vi "Section Page.vi"(8 "error in (no error)":errorcluster, 11 "Node Ptr":T1 format="%.0x") -> (0 "error out":errorcluster)   [LabVIEW 2019, in "Ghost Bus Addon System Explorer.lvlib"]
uses:
  Ghost Bus Addon System Explorer.lvlib
  <vilib>/NI VeriStand/Custom Device API/Custom Device API.lvlib
  Addon Shared/SubVIs/GUID Lookup.vi
  Addon Shared/Ghost Bus Addon Shared.lvlib
  <vilib>/NI VeriStand/Custom Device API/Custom Device Item Ref.ctl
panel:
  in  "SHDocVw.IWebBrowser2":refnum<k7>(container)
types:
  T1 = typedef "Custom Device API.lvlib/Custom Device Item Ref.ctl" = u64
  T2 = typedef "Custom Device API.lvlib/Custom Device Item Info.ctl" = cluster{"Name":string, "Is Channel":bool, "GUID":string, "Is Waveform":bool}
  T3 = typedef "Custom Device API.lvlib/Custom Device Commands.ctl" = enum16{"Default", "Item renamed", "Shutdown", "Dynamic button pressed"}
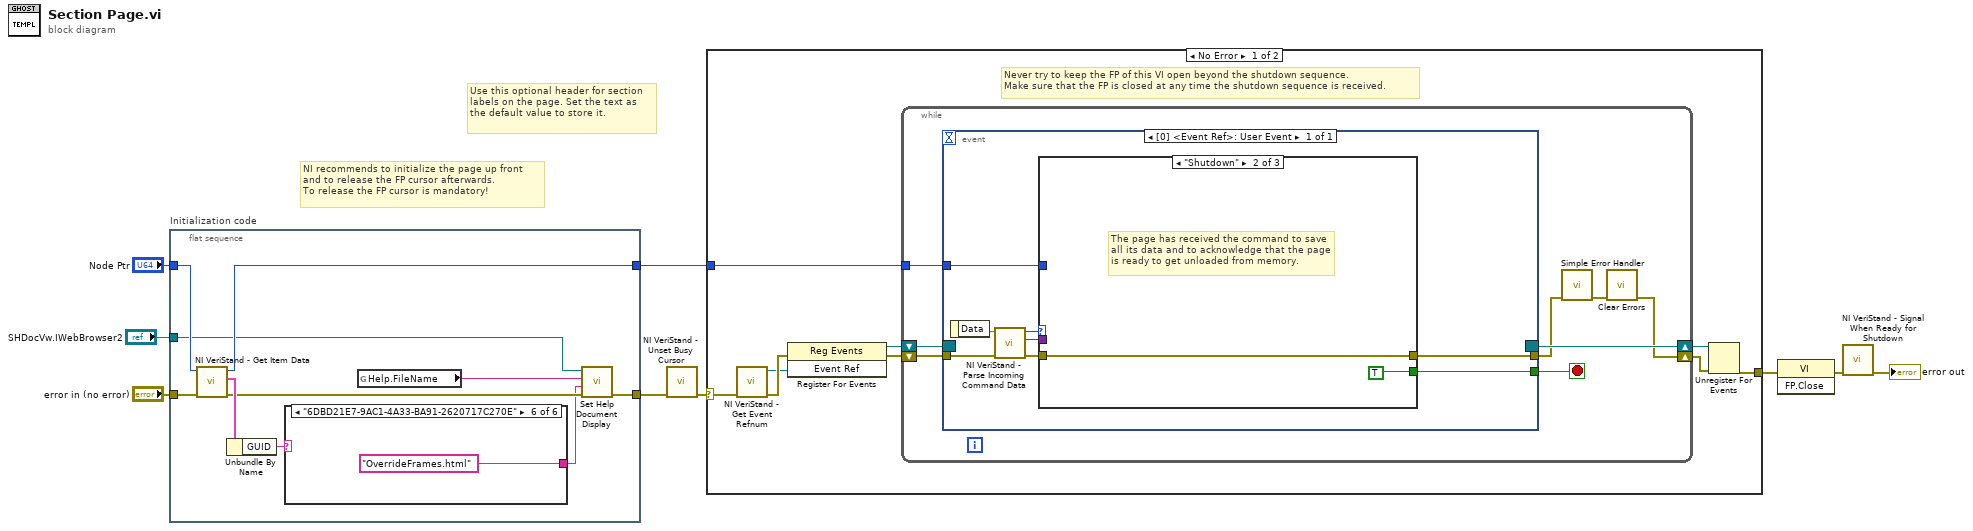
[diagram p0: block diagram]
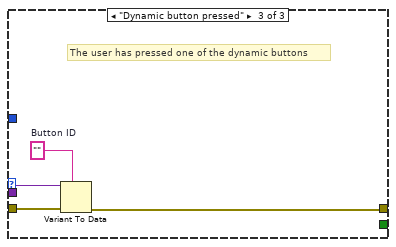
[diagram p3: hidden frame]
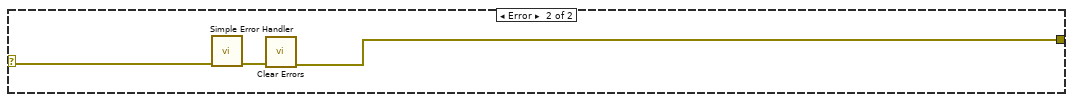
[diagram p4: hidden frame]
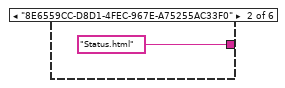
[diagram p6: hidden frame]
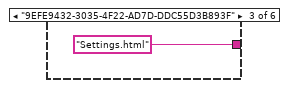
[diagram p7: hidden frame]
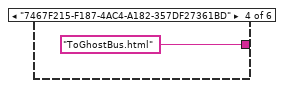
[diagram p8: hidden frame]
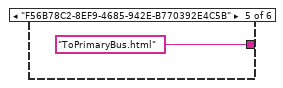
[diagram p9: hidden frame]
diagram:
  # "Use this optional header for section labels on the page. Set the text as the default value to store it."
  # "NI recommends to initialize the page up front\nand to release the FP cursor afterwards.\nTo release the FP cursor is mandatory!"
  n1 = flat-sequence "Initialization code" {
    tunnel: "error in (no error)" -> [w17]
    tunnel: "Node Ptr" -> [w19]
    tunnel: [w13] -> w5
    tunnel: [w18] -> w2
    tunnel: "SHDocVw.IWebBrowser2" -> [w11]
    frame #0 {
      n2 = call <vilib>:"NI VeriStand - Get Item Data.vi"("error in (no error)"=w17, "Item Ref in"=w19) -> ("error out"=w14:errorcluster, "Item Info"=w16:T2, "Item Ref out"=w18:T1)  [unwired: 6 in, 1 out]
      n3 = Unbundle By Name(w16) -> ("GUID"=w15:string)
      n4 = case shown="\"6DBD21E7-9AC1-4A33-BA91-2620717C270E\"" w15 {
        tunnel: [_ "Status.html" ("HTML File") "Settings.html" ("HTML File") "ToGhostBus.html" ("HTML File") "ToPrimaryBus.html" ("HTML File") "OverrideFrames.html" ("HTML File")] -> w12
        frame Default {
        }
        frame "8E6559CC-D8D1-4FEC-967E-A75255AC33F0" {
        }
        frame "9EFE9432-3035-4F22-AD7D-DDC55D3B893F" {
        }
        frame "7467F215-F187-4AC4-A182-357DF27361BD" {
        }
        frame "F56B78C2-8EF9-4685-942E-B770392E4C5B" {
        }
        frame "6DBD21E7-9AC1-4A33-BA91-2620717C270E" {
        }
      }
      n5 = global read "GUID Lookup.vi" "Help.FileName"() -> (w10:string)
      n6 = call "Set Help Document Display.vi"("error in (no error)"=w14, "HTML File"=w12, "Main CHM File"=w10, "SHDocVw.IWebBrowser2"=w11) -> ("error out"=w13:errorcluster)  [unwired: 7 in]
    }
  }
  n7 = call <vilib>:"NI VeriStand - Unset Busy Cursor.vi"("error in (no error)"=w5) -> ("error out"=w4:errorcluster)  [unwired: 10 out]
  n8 = case shown="No Error" w4 {
    selector: w4 -> [w25 w59]
    tunnel: [w30 w57] -> w9
    tunnel: w2 -> [w26 _]
    frame No Error {
      # "Never try to keep the FP of this VI open beyond the shutdown sequence.\nMake sure that the FP is closed at any time the shutdown sequence is received."
      n9 = call <vilib>:"NI VeriStand - Get Event Refnum.vi"("error in (no error)"=w25) -> ("error out"=w33:errorcluster, "Event Ref"=w29:refnum<user-event>)  [unwired: 9 out]
      n10 = register-events(error in=w33, w29) -> (reference out=w27:refnum<event-registration>, error out=w28:errorcluster)  [unwired: 1 in]
      n11 = while {
        tunnel: w26 -> [w37]
        shift-right: [w34] -> w31
        shift-left: w28 -> [w40]
        shift-right: [w41] -> w32
        shift-left: w27 -> [w39]
        stop <- w38 stop-if-true
        n12 = event shown="[0] <Event Ref>: User Event" {
          selector: w39 -> [_]
          dyn-events: [_] -> w41
          timeout: _ -> [_]
          tunnel: w40 -> [w49]
          tunnel: [w45] -> w38
          tunnel: [w44] -> w36
          tunnel: w37 -> [w43]
          event User Event {
            n13 = event-data() -> ("Data"=w48:string)  [unwired: 1 out]
            n14 = call <vilib>:"NI VeriStand - Parse Incoming Command Data.vi"("error in (no error)"=w49, "Incoming data"=w48) -> ("error out"=w47:errorcluster, "Outgoing data"=w42:variant, "Action"=w46:T3)  [unwired: 7 out]
            n15 = case shown="\"Shutdown\"" w46 {
              tunnel: w47 -> [w50 w51 w56]
              tunnel: [_ TRUE _] -> w45
              tunnel: [w50 w51 w53] -> w44
              tunnel: w43 -> [_ _ _]
              tunnel: w42 -> [_ _ w55]
              frame "Default", Default {
              }
              frame "Shutdown" {
                # "The page has received the command to save all its data and to acknowledge that the page is ready to get unloaded from memory."
              }
              frame "Dynamic button pressed" {
                w54 = ""  # Button ID
                # "The user has pressed one of the dynamic buttons"
                n16 = Variant To Data(error in=w56, type=w54, Variant=w55) -> (error out=w53:errorcluster)  [unwired: 1 out]
              }
            }
          }
        }
        n17 = call <vilib>:"Simple Error Handler.vi"("error in (no error)"=w36) -> ("error out"=w35:errorcluster)  [unwired: 1 in, 7 out]
        n18 = call <vilib>:"Clear Errors.vi"("error in (no error)"=w35) -> ("error out"=w34:errorcluster)  [unwired: 1 in, 5 out]
      }
      n19 = Unregister For Events(event registration refnum=w32, error in=w31) -> (error out=w30:errorcluster)
    }
    frame Error {
      n20 = call <vilib>:"Simple Error Handler.vi"("error in (no error)"=w59) -> ("error out"=w58:errorcluster)  [unwired: 1 in, 7 out]
      n21 = call <vilib>:"Clear Errors.vi"("error in (no error)"=w58) -> ("error out"=w57:errorcluster)  [unwired: 1 in, 5 out]
    }
  }
  n22 = invoke class="VI" method="FP.Close"(error in=w9) -> (error out=w8:errorcluster)  [unwired: 2 in, 2 out]
  n23 = call <vilib>:"NI VeriStand - Signal When Ready for Shutdown.vi"("error in (no error)"=w8) -> ("error out"=→"error out":errorcluster)  [unwired: 10 out]
